vi "laserON-OFF.vi"(11 "ON-OFF":bool) -> ()   [LabVIEW 2018]
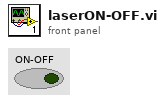
[diagram p1: front panel]
types:
  T1 = cluster{"Instruct Data":i32, "Op Code":i32, "Flags":bool[], "Comments":string, "Time":dbl}
  T2 = cluster{"Instruct Data":i32, "Op Code":i32, "Flags":bool[], "Comments":string, "Time":dbl}[]
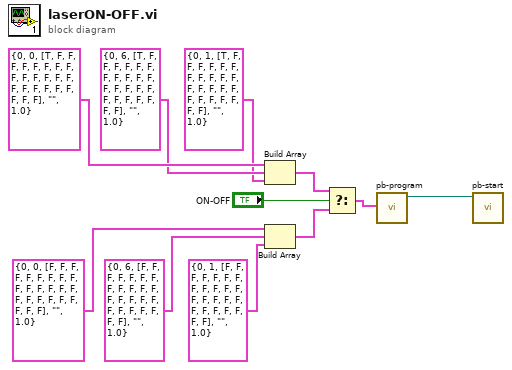
[diagram p0: block diagram]
diagram:
  n1 = Build Array(T1 {"Instruct Data"=0, "Op Code"=0, "Flags"=[TRUE, FALSE, FALSE, FALSE, FALSE, FALSE, FALSE, FALSE, FALSE, FALSE, FALSE, FALSE, FALSE, FALSE, FALSE, FALSE, FALSE, FALSE, FALSE, FALSE, FALSE, FALSE, FALSE, FALSE], "Comments"="", "Time"=1.0} ("PB Instruction"), T1 {"Instruct Data"=0, "Op Code"=6, "Flags"=[TRUE, FALSE, FALSE, FALSE, FALSE, FALSE, FALSE, FALSE, FALSE, FALSE, FALSE, FALSE, FALSE, FALSE, FALSE, FALSE, FALSE, FALSE, FALSE, FALSE, FALSE, FALSE, FALSE, FALSE], "Comments"="", "Time"=1.0} ("PB Instruction"), T1 {"Instruct Data"=0, "Op Code"=1, "Flags"=[TRUE, FALSE, FALSE, FALSE, FALSE, FALSE, FALSE, FALSE, FALSE, FALSE, FALSE, FALSE, FALSE, FALSE, FALSE, FALSE, FALSE, FALSE, FALSE, FALSE, FALSE, FALSE, FALSE, FALSE], "Comments"="", "Time"=1.0} ("PB Instruction")) -> (w3:T2)
  n2 = Build Array(T1 {"Instruct Data"=0, "Op Code"=0, "Flags"=[FALSE, FALSE, FALSE, FALSE, FALSE, FALSE, FALSE, FALSE, FALSE, FALSE, FALSE, FALSE, FALSE, FALSE, FALSE, FALSE, FALSE, FALSE, FALSE, FALSE, FALSE, FALSE, FALSE, FALSE], "Comments"="", "Time"=1.0} ("PB Instruction"), T1 {"Instruct Data"=0, "Op Code"=6, "Flags"=[FALSE, FALSE, FALSE, FALSE, FALSE, FALSE, FALSE, FALSE, FALSE, FALSE, FALSE, FALSE, FALSE, FALSE, FALSE, FALSE, FALSE, FALSE, FALSE, FALSE, FALSE, FALSE, FALSE, FALSE], "Comments"="", "Time"=1.0} ("PB Instruction"), T1 {"Instruct Data"=0, "Op Code"=1, "Flags"=[FALSE, FALSE, FALSE, FALSE, FALSE, FALSE, FALSE, FALSE, FALSE, FALSE, FALSE, FALSE, FALSE, FALSE, FALSE, FALSE, FALSE, FALSE, FALSE, FALSE, FALSE, FALSE, FALSE, FALSE], "Comments"="", "Time"=1.0} ("PB Instruction")) -> (w2:T2)
  n3 = Select(t=w3, s="ON-OFF", f=w2) -> (s? t:f=w1:T2)
  n4 = call "pb-program.vi"("Commands"=w1) -> ("path out"=w10:path)  [unwired: 10 in]
  n5 = call "pb-start.vi"("path in"=w10) -> ()  [unwired: 10 in, 1 out]
